vi "PicoScope4000aExampleBlockMultiUnit.vi"() -> ()   [LabVIEW 2010]
doc: "This example demonstrates how to use the PicoScope Labview library to collect data using block mode."
uses:
  shared/PicoBuffers.ctl
  shared/Buffer and Transfer Settings.ctl
  shared/Acquisition Settings.ctl
  PicoScope4000aLib/PicoScope4000aAnalogChannelSettings.ctl
panel:
  out "Properties panel":T1(array[cluster]) {"Sample Frequency" format="%.3p"; "Sample Rate" format="%.3p"; "Max Samples Available" format="%.3p"; "Number of Samples" format="%.3p"; "Total Capture Time (sec)" format="%.3p"; "Max Total Capture Time Available (sec)" format="%.3p"}
  out "Device Info":T2(array[cluster])
  in  "Scope Index":i32
  out "Scope \"N\"":cluster{i32, dbl, "Data":dbl[]}[](graph)
  out "Overflow":i16[](array[numeric])
  in  "Resolution":u32(ring)=1 items=["8-bit", "12-bit", "14-bit"]
  in  "Trigger Settings":T3={"Trigger Enabled"=FALSE, "Trigger Source"=enum."Channel A", "Trigger Threshold (Volts/Probe units)"=0.0, "Trigger Direction"=2, "Trigger Delay (samples)"=0, "Auto Trigger Time (ms)"=1000} {"Trigger Direction" items=["Rising"=2, "Falling"=3]}
  in  "Apply Settings":bool
  in  "Channel A Settings":T4={"Enabled"=TRUE, "Coupling"=1, "Range"=8, "Analogue Offset"=0.0, "Bandwidth Limit"=0} {"Bandwidth Limit" items=["Full", "20kHz", "100kHz", "1MHz"]; "Range" items=["10 mV", "20 mV", "50 mV", "100 mV", "200 mV", "500 mV", "1 V", "2 V", "5 V", "10 V", "20 V", "50 V ", "100 V"]; "Coupling" items=["AC", "DC"]}
  out "USB 3.0 device on non-USB 3.0 Port":bool=TRUE
  out "USB Powered":bool=TRUE
  out "error out":errorcluster
  in  "Buffer and Transfer Settings":T5={"startIndex"=0, "Samples"=5000000, "Down Sample Ratio"=1, "Down-Sample Mode"=0} {"Down-Sample Mode" items=["RAW none"=2147483648, "None"=0, "Aggregate"=1, "Decimate"=2, "Average"=4]; "Down Sample Ratio" step=1; "Samples" format="%_6p"}
  in  "Acquisition Settings":T6={"preTriggerSamples"=0, "postTriggerSamples"=5000000, "timebase"=5} {"postTriggerSamples" format="%_6p"; "preTriggerSamples" format="%_6p"}
  in  "stop":bool
  in  "Serial Numbers":string[](array[string])
  in  "Use Serial Numbers":bool
  in  "error in (no error)":errorcluster
  # "Bit 0 = ChA"
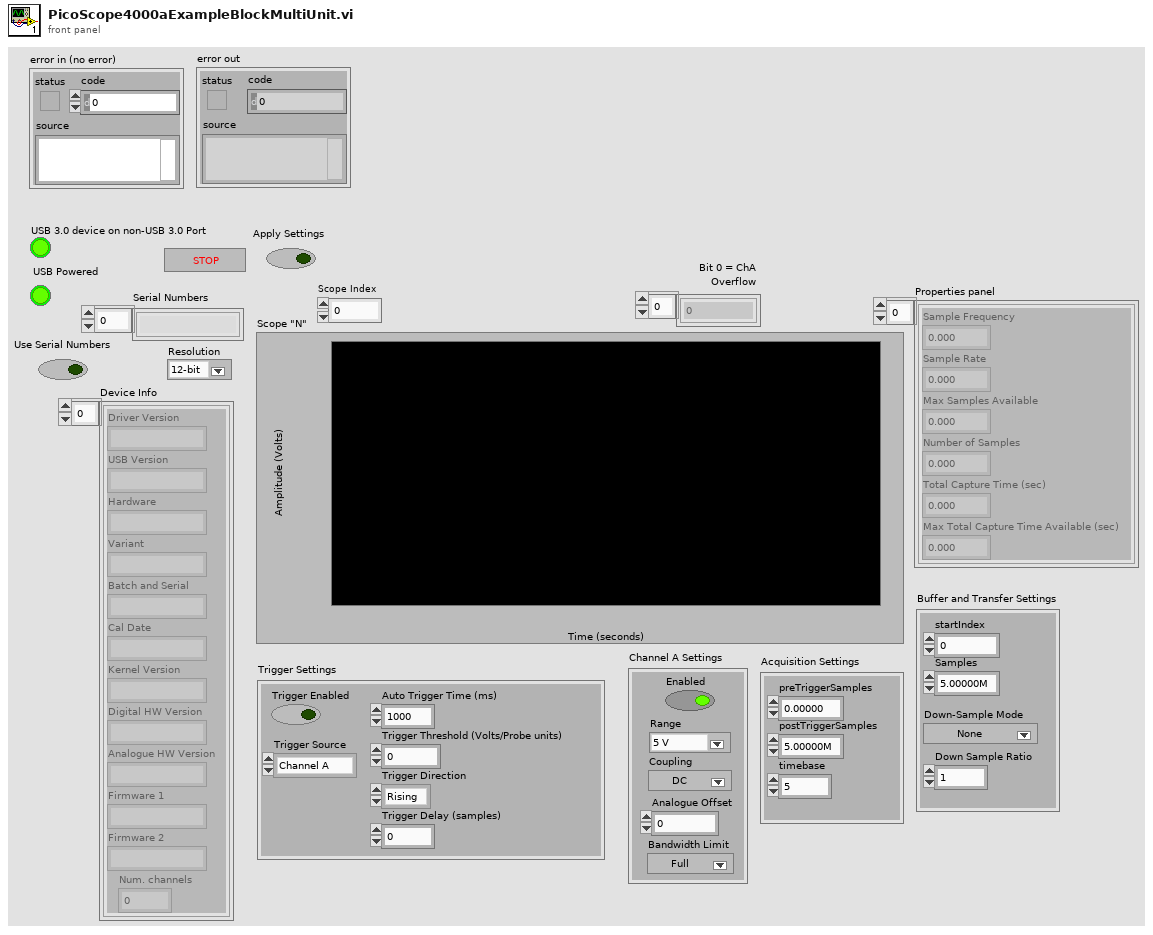
[diagram p1: front panel]
types:
  T1 = cluster{"Sample Frequency":dbl, "Sample Rate":dbl, "Max Samples Available":u64, "Number of Samples":u64, "Total Capture Time (sec) ":dbl, "Max Total Capture Time Available (sec)":dbl}[]
  T2 = cluster{"Driver Version":string, "USB Version":string, "Hardware":string, "Variant":string, "Batch and Serial":string, "Cal Date":string, "Kernel Version":string, "Digital HW Version":string, "Analogue HW Version":string, "Firmware 1":string, "Firmware 2":string, "Num. channels":i16}[]
  T3 = cluster{"Trigger Enabled":bool, "Trigger Source":enum16{"Channel A", "Channel B", "Channel C", "Channel D", "Channel E", "Channel F", "Channel G", "Channel H"}, "Trigger Threshold (Volts/Probe units)":dbl, "Trigger Direction":u16, "Trigger Delay (samples)":u32, "Auto Trigger Time (ms)":i16}
  T4 = typedef "PicoScope4000aAnalogChannelSettings.ctl" = cluster{"Enabled":bool, "Coupling":i16, "Range":u32, "Analogue Offset":sgl, "Bandwidth Limit":u32}
  T5 = typedef "Buffer and Transfer Settings.ctl" = cluster{"startIndex":u64, "Samples":u64, "Down Sample Ratio":u64, "Down-Sample Mode":u32}
  T6 = typedef "Acquisition Settings.ctl" = cluster{"preTriggerSamples":u64, "postTriggerSamples":u64, "timebase":u32}
  T7 = typedef "PicoBuffers.ctl" = cluster{"Max Buffer Pointers":u64[][][], "Min Buffer Pointers":u64[][][], "StreamingDataInfo":cluster{"Channel":u32, "Down-Sample Mode":u32, "PICO_DATA_TYPE":enum32{"PICO_INT8_T", "PICO_INT16_T", "PICO_INT32_T", "PICO_UINT32_T", "PICO_INT64_T", ""}, "Samples":i32, "bufferIndex":u64, "startIndex":i32, "overflow":i16}[][]}
  T8 = cluster{"Driver Version":string, "USB Version":string, "Hardware":string, "Variant":string, "Batch and Serial":string, "Cal Date":string, "Kernel Version":string, "Digital HW Version":string, "Analogue HW Version":string, "Firmware 1":string, "Firmware 2":string, "Num. channels":i16}
  T9 = cluster{"Sample Frequency":dbl, "Sample Rate":dbl, "Max Samples Available":u64, "Number of Samples":u64, "Total Capture Time (sec) ":dbl, "Max Total Capture Time Available (sec)":dbl}
  T10 = cluster{"Channel A Buffer":i16[], "Channel B Buffer":i16[], "Channel C Buffer":i16[], "Channel D Buffer":i16[], "Channel E Buffer":i16[], "Channel F Buffer":i16[], "Channel G Buffer":i16[], "Channel H Buffer":i16[], "Port 0 Buffer":i16[], "Port 1 Buffer":i16[]}[]
  T11 = cluster{"Channel A Buffer":i16[], "Channel B Buffer":i16[], "Channel C Buffer":i16[], "Channel D Buffer":i16[], "Channel E Buffer":i16[], "Channel F Buffer":i16[], "Channel G Buffer":i16[], "Channel H Buffer":i16[], "Port 0 Buffer":i16[], "Port 1 Buffer":i16[]}
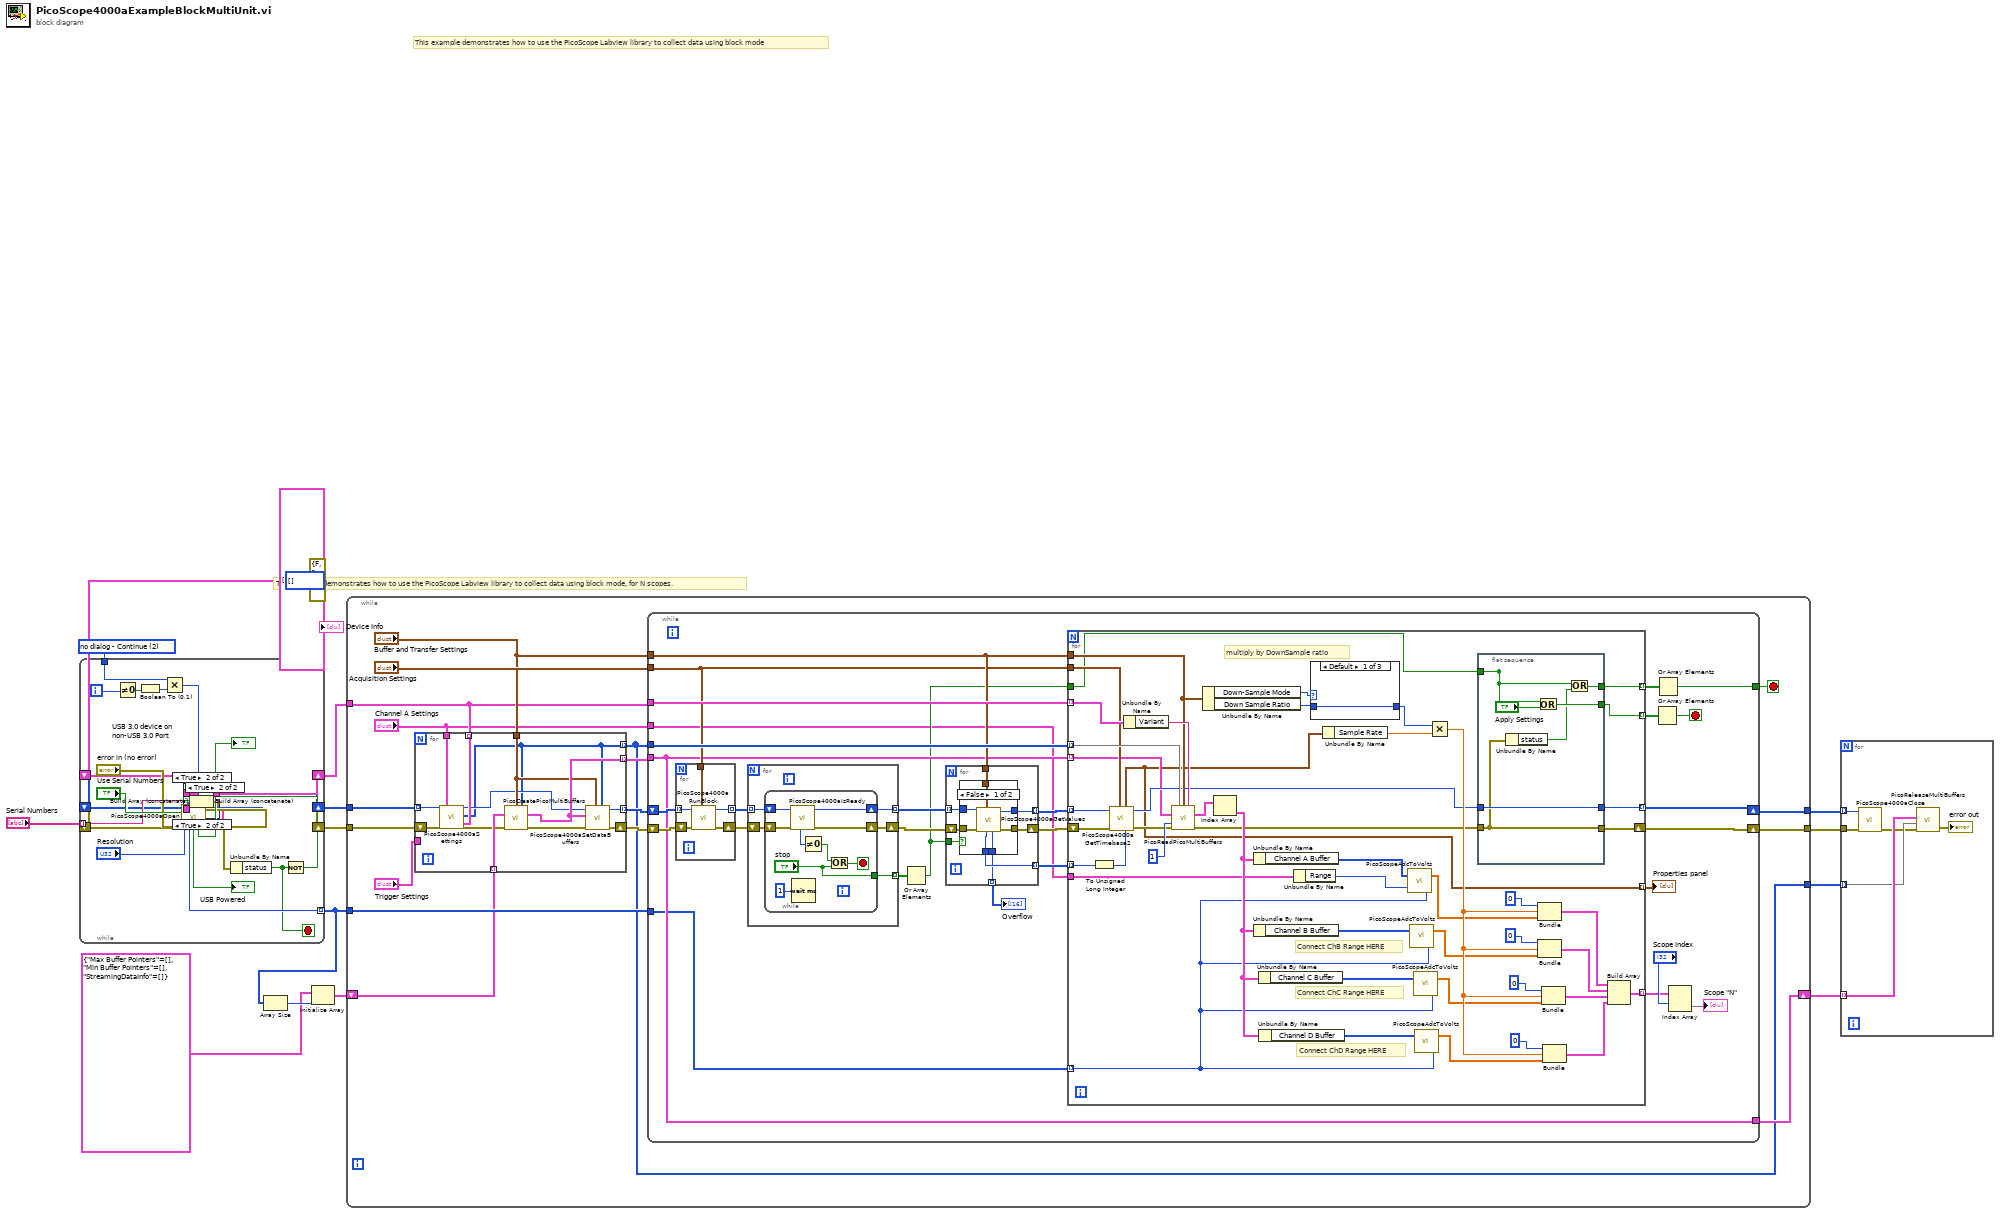
[diagram p0: block diagram]
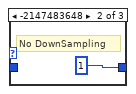
[diagram p5: hidden frame]
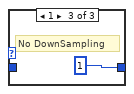
[diagram p6: hidden frame]
diagram:
  w10 = u16 2 items=["Dialog On Error", "no dialog - CloseUnit and Stop", "no dialog - Continue", "no dialog - Stop"] ("Mode")
  # "This example demonstrates how to use the PicoScope Labview library to collect data using block mode, for N scopes."
  # "This example demonstrates how to use the PicoScope Labview library to collect data using block mode"
  n1 = while {
    tunnel: [w39] -> w7 mode=indexing
    tunnel: w10 -> [w33]
    tunnel: "Serial Numbers" -> [w27] mode=indexing
    shift-right: [w21] -> w13
    shift-left: T2 [] ("Array") -> [w22]
    shift-right: [w19] -> w12
    shift-left: i16[] [] ("Array") -> [w20]
    shift-right: [w17] -> w11
    shift-left: errorcluster {"status"=FALSE, "code"=0, "source"=""} ("error out 2") -> [w18]
    i -> [w32]
    stop <- w29 stop-if-true
    n2 = Not Equal To 0?(x=w32) -> (x != 0?=w35:bool)
    n3 = Boolean To (0,1)(Boolean=w35) -> (0, 1=w34:i16)
    n4 = Multiply(x=w33, y=w34) -> (x*y=w31:u16)
    n5 = call "PicoScope4000aOpen.vi"("Serial Number"=w27, "Mode"=w31, "Use Serial Number"="Use Serial Numbers", "Resolution"="Resolution", "error in (no error)"="error in (no error)") -> ("handle"=w24:i16, "Unit Info"=w23:T8, "Max ADC value"=w39:i16, "USB powered"=→"USB Powered":bool, "USB 3.0 on non-USB 3.0 port"=→"USB 3.0 device on non-USB 3.0 Port":bool, "error out"=w26:errorcluster)  [unwired: 3 in, 2 out]
    n6 = Unbundle By Name(w26) -> ("status"=w29:bool)
    n7 = Not(x=w29) -> (.not. x?=w30:bool)
    n8 = case shown="True" w30 {
      tunnel: w18 -> [w40 _]
      tunnel: w26 -> [_ w41]
      tunnel: [w40 w41] -> w17
      frame False {
      }
      frame True {
      }
    }
    n9 = case shown="True" w30 {
      tunnel: w20 -> [w42 w44]
      tunnel: w24 -> [_ w43]
      tunnel: [w42 w45] -> w19
      frame False {
      }
      frame True {
        n10 = Build Array (concatenate)(w44, w43) -> (w45:i16[])
      }
    }
    n11 = case shown="True" w30 {
      tunnel: w22 -> [w46 w48]
      tunnel: w23 -> [_ w47]
      tunnel: [w46 w49] -> w21
      frame False {
      }
      frame True {
        n12 = Build Array (concatenate)(w48, w47) -> (w49:T2)
      }
    }
  }
  n13 = Array Size(array=w7) -> (size(s)=w9:i32)
  n14 = Initialize Array(T7 {"Max Buffer Pointers"=[], "Min Buffer Pointers"=[], "StreamingDataInfo"=[]} ("Data Pointers"), w9) -> (w8:T7[])
  n15 = while {
    tunnel: w12 -> [w54]
    tunnel: w7 -> [w63]
    tunnel: [w51] -> w16
    tunnel: w11 -> [w65]
    tunnel: [w62] -> w15
    tunnel: [w60] -> w14
    tunnel: w13 -> [w52]
    shift-right: [w55] -> w5
    shift-left: w8 -> [w53]
    stop <- w61 stop-if-true
    n16 = for {
      tunnel: [w78] -> w66 mode=indexing
      tunnel: [w67] -> w51 mode=indexing
      tunnel: "Channel A Settings" -> [w77]
      tunnel: [w75] -> w58 mode=indexing
      tunnel: "Buffer and Transfer Settings" -> [w74]
      tunnel: "Trigger Settings" -> [_]
      shift-right: [w76] -> w59
      shift-left: w65 -> [w70]
      tunnel: w54 -> [w71] mode=indexing
      tunnel: w53 -> [w73] mode=indexing
      tunnel: w52 -> [w72] mode=indexing
      n17 = call "PicoScope4000aSettings.vi"("handle in"=w71, "error in"=w70, "Channel A Settings"=w77, "Unit Info"=w72) -> ("handle out"=w69:i16, "Enabled array"=w67:i16[], "error out"=w68:errorcluster)  [unwired: 13 in]
      n18 = call "PicoCreatePicoMultiBuffers.vi"("Buffer and Transfer Settings"=w74, "enabled array"=w67, "Data Pointers In"=w73, "error in (no error)"=w68) -> ("Data Pointers"=w78:T7, "error out"=w79:errorcluster)  [unwired: 10 in]
      n19 = call "PicoScope4000aSetDataBuffers.vi"("enabled array"=w67, "Buffer and Transfer Settings"=w74, "error in (no error)"=w79, "Data Pointers In"=w78, "handle in"=w69) -> ("error out"=w76:errorcluster, "handle out"=w75:i16)  [unwired: 5 in]
    }
    n20 = while {
      tunnel: w66 -> [w93]
      tunnel: "Buffer and Transfer Settings" -> [w98]
      tunnel: w51 -> [w106]
      tunnel: "Acquisition Settings" -> [w94]
      tunnel: w63 -> [w90]
      tunnel: w52 -> [w105]
      tunnel: [w87] -> w61
      shift-right: [w104] -> w62
      shift-left: w59 -> [w99]
      shift-right: [w103] -> w60
      shift-left: w58 -> [w100]
      tunnel: [w93] -> w55
      tunnel: "Channel A Settings" -> [w89]
      stop <- w84 stop-if-true
      n21 = for {
        tunnel: [w200] -> w107 mode=indexing
        tunnel: w100 -> [w199] mode=indexing
        tunnel: w94 -> [w197]
        shift-right: [w201] -> w108
        shift-left: w99 -> [w198]
        n22 = call "PicoScope4000aRunBlock.vi"("Acquisition Settings"=w197, "error in (no error)"=w198, "handle in"=w199) -> ("error out"=w201:errorcluster, "handle out"=w200:i16)  [unwired: 5 in, 2 out]
      }
      n23 = for {
        tunnel: w107 -> [w186] mode=indexing
        tunnel: [w185] -> w102 mode=indexing
        tunnel: [w183] -> w92 mode=indexing
        shift-right: [w184] -> w101
        shift-left: w108 -> [w187]
        n24 = while {
          shift-right: [w195] -> w184
          shift-left: w187 -> [w196]
          shift-right: [w194] -> w185
          shift-left: w186 -> [w193]
          tunnel: ["stop"] -> w183
          stop <- w190 stop-if-true
          n25 = call "PicoScope4000aIsReady.vi"("error in (no error)"=w196, "handle in"=w193) -> ("error out"=w195:errorcluster, "handle out"=w194:i16, "ready"=w192:i16)  [unwired: 7 in]
          n26 = Wait (ms)(milliseconds to wait=u32 1) -> ()  [unwired: 1 out]
          n27 = Not Equal To 0?(x=w192) -> (x != 0?=w191:bool)
          n28 = Or(x=w191, y="stop") -> (x .or. y?=w190:bool)
        }
      }
      n29 = Or Array Elements(Boolean array=w92) -> (logical OR=w91:bool)
      n30 = for {
        tunnel: w102 -> [w173] mode=indexing
        tunnel: w98 -> [w171]
        tunnel: [w170] -> w97 mode=indexing
        tunnel: [w168] -> w95 mode=indexing
        tunnel: w91 -> [w167]
        shift-right: [w169] -> w96
        shift-left: w101 -> [w172]
        tunnel: [w166] -> w88 mode=indexing
        n31 = case shown="False" w167 {
          tunnel: w172 -> [w180 w181]
          tunnel: w173 -> [w179 w182]
          tunnel: [w178 w182] -> w168
          tunnel: [w177 w181] -> w169
          tunnel: w171 -> [w176 _]
          tunnel: [w175 _] -> w166
          tunnel: [w174 _] -> w170
          frame False {
            n32 = call "PicoScope4000aGetValues.vi"("Buffer and Transfer Settings"=w176, "error in (no error)"=w180, "handle in"=w179) -> ("error out"=w177:errorcluster, "handle out"=w178:i16, "overflow"=w175:i16, "noOfSamples"=w174:u64)  [unwired: 5 in]
          }
          frame True {
          }
        }
      }
      "Overflow" <- w88
      n33 = for {
        tunnel: w106 -> [w150] mode=indexing
        tunnel: w105 -> [w147] mode=indexing
        tunnel: [w138] -> w81 mode=indexing
        tunnel: [w123] -> w103 mode=indexing
        tunnel: w98 -> [w122]
        tunnel: w97 -> [w111] mode=indexing
        tunnel: w95 -> [w119] mode=indexing
        tunnel: w94 -> [w117]
        tunnel: w93 -> [w116] mode=indexing
        shift-right: [w126] -> w104
        shift-left: w96 -> [w120]
        tunnel: w90 -> [w114] mode=indexing
        tunnel: w89 -> [w113]
        tunnel: w91 -> [w115]
        tunnel: [w124] -> w86 mode=indexing
        tunnel: [w110] -> w85 mode=indexing
        tunnel: [w109] -> w80 mode=indexing
        # "Connect ChB Range HERE"
        # "Connect ChD Range HERE"
        # "Connect ChC Range HERE"
        # "multiply by DownSample ratio"
        n34 = To Unsigned Long Integer(number=w111) -> (unsigned 32bit integer=w112:u32)
        n35 = call "PicoScope4000aGetTimebase2.vi"("Number of Samples"=w112, "Acquisition Settings"=w117, "error in (no error)"=w120, "handle in"=w119) -> ("error out"=w121:errorcluster, "handle out"=w118:i16, "Properties Panel"=w109:T9)  [unwired: 5 in]
        n36 = Unbundle By Name(w147) -> ("Variant"=w148:string)
        n37 = call "PicoReadPicoMultiBuffers.vi"("enabled array"=w150, "Buffer and Transfer Settings"=w122, "Variant"=w148, "Data Pointers"=w116, "No of Buffers"=1, "error in (no error)"=w121) -> ("MultiBuffers (Max or non-aggregated)"=w155:T10, "error out"=w125:errorcluster)  [unwired: 7 in, 1 out]
        n38 = Unbundle By Name(w122) -> ("Down-Sample Mode"=w153:u32, "Down Sample Ratio"=w154:u64)
        n39 = Index Array(array=w155) -> (element=w127:T11)  [unwired: 1 in]
        n40 = Unbundle By Name(w127) -> ("Channel A Buffer"=w136:i16[])
        n41 = Unbundle By Name(w127) -> ("Channel B Buffer"=w142:i16[])
        n42 = Unbundle By Name(w127) -> ("Channel C Buffer"=w134:i16[])
        n43 = Unbundle By Name(w127) -> ("Channel D Buffer"=w130:i16[])
        n44 = Unbundle By Name(w113) -> ("Range"=w144:u32)
        n45 = case shown="Default" w153 {
          tunnel: [w163 u64 1 ("Down Sample Ratio") u64 1 ("Down Sample Ratio")] -> w151
          tunnel: w154 -> [w163 _ _]
          frame Default {
          }
          frame -2147483648 {
            # "No DownSampling"
          }
          frame 1 {
            # "No DownSampling"
          }
        }
        n46 = Unbundle By Name(w109) -> ("Sample Rate"=w149:dbl)
        n47 = call "PicoScopeAdcToVolts.vi"("Max_adc"=w114, "Range Index"=w144, "Data"=w136) -> ("Data"=w137:dbl[])
        n48 = call "PicoScopeAdcToVolts.vi"("Max_adc"=w114, "Data"=w142) -> ("Data"=w141:dbl[])  [unwired: 1 in]
        n49 = call "PicoScopeAdcToVolts.vi"("Max_adc"=w114, "Data"=w134) -> ("Data"=w133:dbl[])  [unwired: 1 in]
        n50 = call "PicoScopeAdcToVolts.vi"("Max_adc"=w114, "Data"=w130) -> ("Data"=w129:dbl[])  [unwired: 1 in]
        n51 = Multiply(x=w151, y=w149) -> (x*y=w152:dbl)
        n52 = flat-sequence {
          tunnel: [w162] -> w110
          tunnel: [w156] -> _
          tunnel: [w159] -> w124
          tunnel: w118 -> [w158]
          tunnel: [w158] -> w123
          tunnel: w125 -> [w157]
          tunnel: [w157] -> w126
          tunnel: w115 -> [w156]
          frame #0 {
            n53 = Unbundle By Name(w157) -> ("status"=w160:bool)
            n54 = Or(x=w156, y="Apply Settings") -> (x .or. y?=w162:bool)
            n55 = Or(x=w156, y=w160) -> (x .or. y?=w159:bool)
          }
        }
        n56 = Bundle(0, w152, "Data"=w137) -> (w140:cluster{i32, dbl, "Data":dbl[]})  [unwired: 1 in]
        n57 = Bundle(0, w152, "Data"=w141) -> (w139:cluster{i32, dbl, "Data":dbl[]})  [unwired: 1 in]
        n58 = Bundle(0, w152, "Data"=w133) -> (w132:cluster{i32, dbl, "Data":dbl[]})  [unwired: 1 in]
        n59 = Bundle(0, w152, "Data"=w129) -> (w128:cluster{i32, dbl, "Data":dbl[]})  [unwired: 1 in]
        n60 = Build Array(w140, w139, w132, w128) -> (w138:cluster{i32, dbl, "Data":dbl[]}[])
      }
      "Properties panel" <- w80
      n61 = Or Array Elements(Boolean array=w85) -> (logical OR=w84:bool)
      n62 = Or Array Elements(Boolean array=w86) -> (logical OR=w87:bool)
      n63 = Index Array(array=w81, index (row)="Scope Index") -> (element=→"Scope \"N\"":cluster{i32, dbl, "Data":dbl[]}[])  [unwired: 1 in]
    }
  }
  n64 = for {
    tunnel: w16 -> [w204] mode=indexing
    tunnel: w15 -> [w203]
    tunnel: w14 -> [w206] mode=indexing
    tunnel: w5 -> [w205] mode=indexing
    n65 = call "PicoScope4000aClose.vi"("error in (no error)"=w203, "handle in"=w206) -> ("error out"=w202:errorcluster)  [unwired: 7 in, 1 out]
    n66 = call "PicoReleaseMultiBuffers.vi"("error in (no error)"=w202, "Enabled array"=w204, "Data Pointers"=w205) -> ("error out"=→"error out":errorcluster)  [unwired: 7 in, 1 out]
  }
